vi "SetParam.vi"(8 "error in (no error)":errorcluster caption="entrée d'erreur (pas d'erreur)", 10 "add_dummy_feature":cluster{"value":dbl}={"value"=1.0}, 11 "add_dummy_feature.lvclass":refnum<class "add_dummy_feature.lvclass">) -> (0 "error out":errorcluster caption="sortie d'erreur", 3 "add_dummy_feature.lvclass":refnum<class "add_dummy_feature.lvclass">)   [LabVIEW 2020, in "add_dummy_feature.lvclass"]
doc: "Set Parameters"
uses:
  add_dummy_feature.lvclass
  add_dummy_feature.lvclass/add_dummy_feature.ctl
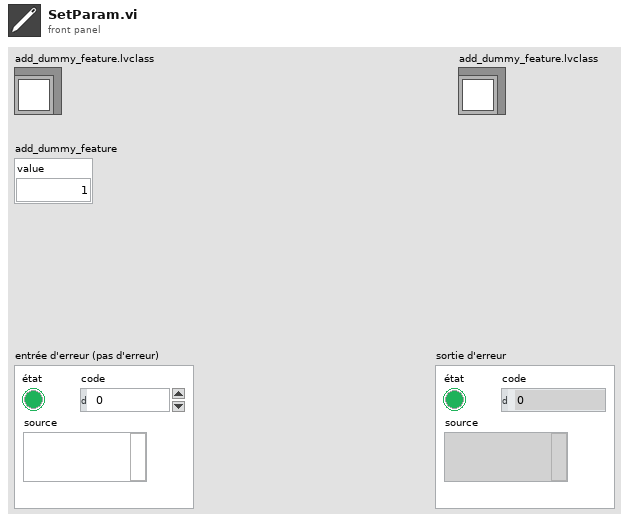
[diagram p1: front panel]
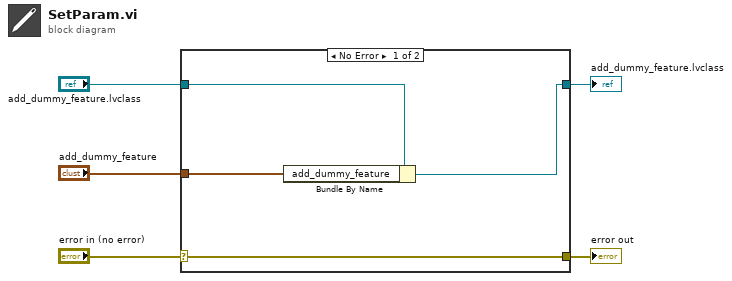
[diagram p0: block diagram]
diagram:
  n1 = case shown="No Error" "error in (no error)" {
    selector: "error in (no error)" -> [w9 w10]
    tunnel: [w9 w10] -> w4
    tunnel: [w7 w11] -> w2
    tunnel: "add_dummy_feature.lvclass" -> [w8 w11]
    tunnel: "add_dummy_feature" -> [w6 _]
    frame No Error {
      n2 = Bundle By Name(cluster=w8, "add_dummy_feature"=w6) -> (w7:refnum<class "add_dummy_feature.lvclass">)
    }
    frame Error {
    }
  }
  "error out" <- w4
  "add_dummy_feature.lvclass" <- w2
